vi "Wrapper_setCorrectForElectricalDarkvi.vi"(9 "enableFlag":bool, 10 "Index in":i32, 11 "Wrapper in":u32) -> (2 "Index out":i32, 3 "Wrapper out":u32)   [LabVIEW 2017]
uses:
  OmniDriver32.dll
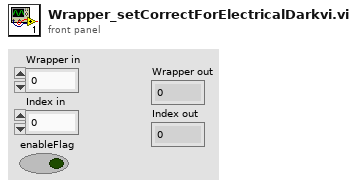
[diagram p1: front panel]
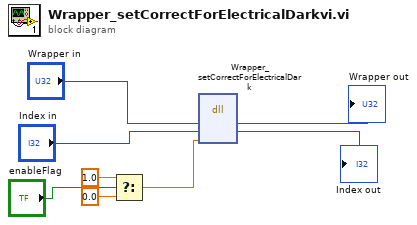
[diagram p0: block diagram]
diagram:
  n1 = Select(t=1.0, s="enableFlag", f=0.0) -> (s? t:f=w4:dbl)
  n2 = dll-call lib="OmniDriver32.dll" fn="Wrapper_setCorrectForElectricalDark" label="Wrapper.getSpectrum"("Wrapper"="Wrapper in", "Index"="Index in", "enableFlag"=w4) -> ("Wrapper"=→"Wrapper out":u32, "Index"=→"Index out":i32)  [unwired: 4 in, 3 out]
